vi "RWPrefFile.vi"(7 "Task":enum16{"Read", "Write"}(ring), 8 "error in (no error)":errorcluster, 11 "Device Name":string) -> (0 "error out":errorcluster, 3 "Device Out":T1={"Name"="", "BaseURL"="", "AppKey"="", "Headers"=["Content-Type:application/json"], "Timeout"=10000, "Identifier"="", "Password"="", "Comments"="", "Handle"=0, "# Handles"=0})   [LabVIEW 2016]
uses:
  Device.ctl
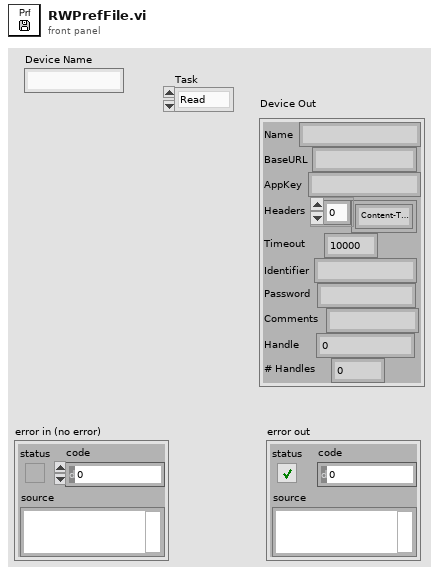
[diagram p1: front panel]
types:
  T1 = typedef "Device.ctl" = cluster{"Name":string, "BaseURL":string, "AppKey":string, "Headers":string[], "Timeout":i32, "Identifier":string, "Password":string, "Comments":string, "Handle":u32, "# Handles":i32}
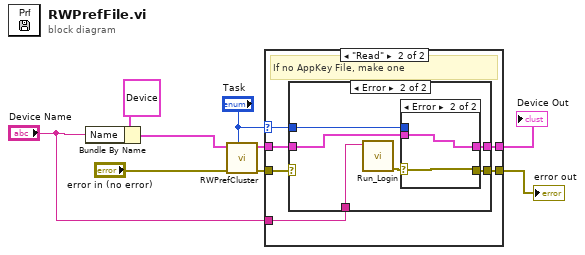
[diagram p0: block diagram]
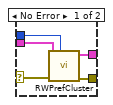
[diagram p4: hidden frame]
diagram:
  n1 = Bundle By Name(cluster=T1 {"Name"="", "BaseURL"="", "AppKey"="", "Headers"=["Content-Type:application/json"], "Timeout"=10000, "Identifier"="", "Password"="", "Comments"="", "Handle"=0, "# Handles"=0} ("Connection in"), "Name"="Device Name") -> (w8:T1)
  n2 = call "RWPrefCluster.vi"("Task"="Task", "error in (no error)"="error in (no error)", "Device In"=w8) -> ("error out"=w5:errorcluster, "Device Out"=w6:T1)  [unwired: 7 in]
  n3 = case shown="\"Read\"" "Task" {
    selector: "Task" -> [_ w12]
    tunnel: w6 -> [w11 w17]
    tunnel: w5 -> [w10 w16]
    tunnel: [w11 w15] -> w4
    tunnel: [w10 w14] -> w3
    tunnel: "Device Name" -> [_ w13]
    frame "Write" {
    }
    frame "Read" {
      # "If no AppKey File, make one"
      n4 = case shown="Error" w16 {
        selector: w16 -> [w18 _]
        tunnel: [w18 w22] -> w14
        tunnel: [w19 w23] -> w15
        tunnel: w17 -> [w19 w24]
        tunnel: w13 -> [_ w25]
        tunnel: w12 -> [_ w21]
        frame No Error {
        }
        frame Error {
          n5 = call "Run_Login.vi"("Device"=w25) -> ("error out"=w20:errorcluster)  [unwired: 10 in]
          n6 = case shown="Error" w20 {
            selector: w20 -> [w26 w31]
            tunnel: w24 -> [w30 w32]
            tunnel: [w29 w32] -> w23
            tunnel: [w28 w31] -> w22
            tunnel: w21 -> [w27 _]
            frame No Error {
              n7 = call "RWPrefCluster.vi"("Task"=w27, "error in (no error)"=w26, "Device In"=w30) -> ("error out"=w28:errorcluster, "Device Out"=w29:T1)  [unwired: 7 in]
            }
            frame Error {
            }
          }
        }
      }
    }
  }
  "error out" <- w3
  "Device Out" <- w4
